vi "Sodium Boiler Model.vi"(5 "Heated Coolant Input (mB/t)":u32, 7 "Superheating Elements":u32=3 min=1 max=70 step=1, 8 "Steam Cavity Height (m)":u32, 9 "Water Cavity Height (m)":u32, 10 "Length (m)":u32=3 min=3 max=18 step=1, 11 "Width (m)":u32=4 min=3 max=18 step=1) -> ()   [LabVIEW 2023]
panel:
  out "Steam Tubes Required":u32=4 min=4 max=18 step=1
  out "Status":bool
  out "Water Demand (mB/t)":u32
  out "Boil Rate (mB/t)":dbl(slide) scale=0.0..9600000.0 scale format="%#_6f"
  out "Sodium Loops Required":u32=4 min=4 max=18 step=1
  out "Water Pipes Required":u32=4 min=4 max=18 step=1
  out "Steam Output (mB/t)":u32
  out "Coolant Output (mB/t)":u32
  out "Maximum Boil Rate (mB/t)":u32=4 min=4 max=18 step=1
  out "Coolant Tank (mB)":u32
  out "Steam Tank (mB)":u32
  out "Pressure Dispersers":u32=4 min=4 max=18 step=1
  out "Heated Coolant Tank (mB)":u32
  out "Water Tank (mB)":u32
  out "Volume (m³)":u32
  out "Height (m)":u32=4 min=4 max=18 step=1
  # "Thermoelectric Boiler Properties"
  # "Note: The boiler's heated coolant tank size must be about twice the size of the\nreactor's coolant tank, with as much coolant buffered in the coolant return tube\nand as much water as the water tank's capacity buffered in the water return tubes."
  # "Thermoelectric Boiler Operation"
  # "+1 for heating elements"
  # "+1 for dispersers"
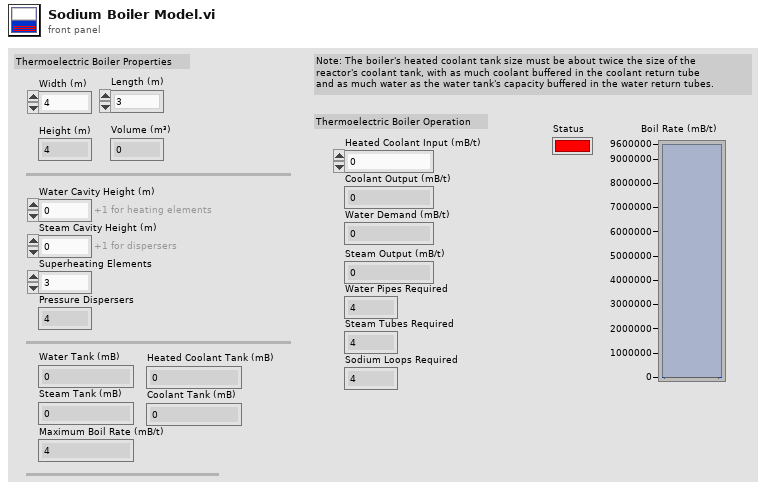
[diagram p1: front panel]
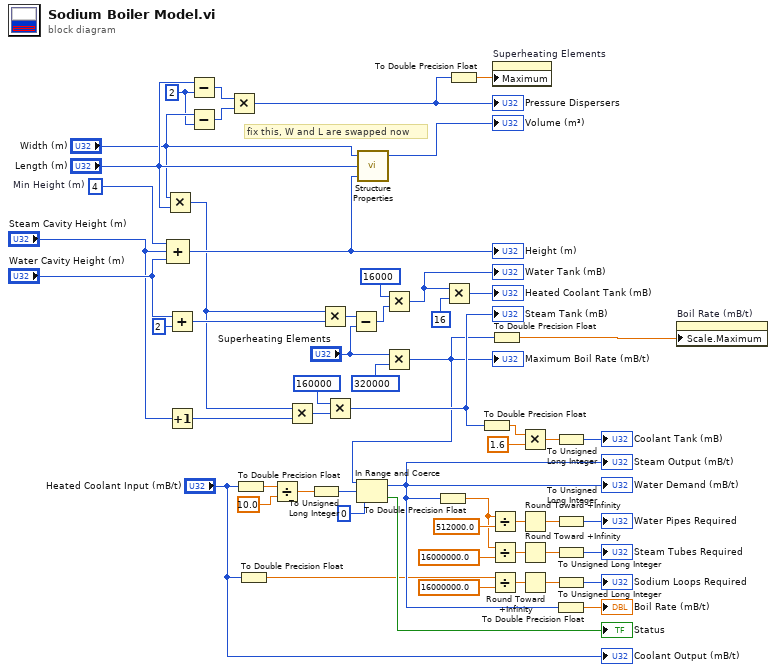
[diagram p0: block diagram]
diagram:
  w46 = u32 2 ("y")
  w55 = u32 4  # Min Height (m)
  # "fix this, W and L are swapped now"
  n1 = Multiply(x="Width (m)", y="Length (m)") -> (x*y=w32:u32)
  n2 = Compound Arithmetic op=ADD(w55, "Steam Cavity Height (m)", "Water Cavity Height (m)") -> (w54:u32)
  "Height (m)" <- w54
  n3 = Add(x="Water Cavity Height (m)", y=u32 2) -> (x+y=w33:u32)
  n4 = Increment(x="Steam Cavity Height (m)") -> (x+1=w31:u32)
  n5 = Subtract(x="Length (m)", y=w46) -> (x-y=w45:u32)
  n6 = Subtract(x="Width (m)", y=w46) -> (x-y=w44:u32)
  n7 = Multiply(x=w45, y=w44) -> (x*y=w2:u32)
  "Pressure Dispersers" <- w2
  n8 = To Double Precision Float(number="Heated Coolant Input (mB/t)") -> (double precision float=w19:dbl)
  n9 = To Double Precision Float(number="Heated Coolant Input (mB/t)") -> (double precision float=w9:dbl)
  n10 = Divide(x=w19, y=10.0) -> (x/y=w20:dbl)
  n11 = Multiply(x=w32, y=w31) -> (x*y=w38:u32)
  n12 = To Unsigned Long Integer(number=w20) -> (unsigned 32bit integer=w17:u32)
  n13 = Multiply(x=w32, y=w33) -> (x*y=w51:u32)
  n14 = Multiply(x=u32 160000 ("y"), y=w38) -> (x*y=w15:u32)
  "Steam Tank (mB)" <- w15
  n15 = Subtract(x=w51, y="Superheating Elements") -> (x-y=w49:u32)
  n16 = call "Structure Properties.vi"("Length"="Width (m)", "Width"="Length (m)", "Height"=w54) -> ("Volume"=→"Volume (m³)":i32)  [unwired: 2 in, 4 out]
  n17 = Multiply(x=u32 16000 ("y"), y=w49) -> (x*y=w43:u32)
  "Water Tank (mB)" <- w43
  n18 = Multiply(x="Superheating Elements", y=u32 320000) -> (x*y=w13:u32)
  "Maximum Boil Rate (mB/t)" <- w13
  n19 = In Range and Coerce(upper limit=w13, x=w17, lower limit=u32 0) -> (coerced(x)=w11:u32, In Range?=→"Status":bool)
  "Steam Output (mB/t)" <- w11
  "Water Demand (mB/t)" <- w11
  n20 = To Double Precision Float(number=w11) -> (double precision float=w3:dbl)
  n21 = Multiply(x=w43, y=u32 16) -> (x*y=→"Heated Coolant Tank (mB)":u32)
  n22 = To Double Precision Float(number=w2) -> (double precision float=w1:dbl)
  n23 = To Double Precision Float(number=w15) -> (double precision float=w14:dbl)
  n24 = Divide(x=w3, y=512000.0) -> (x/y=w27:dbl)
  n25 = Divide(x=w3, y=16000000.0) -> (x/y=w5:dbl)
  n26 = Divide(x=w9, y=16000000.0) -> (x/y=w26:dbl)
  n27 = To Double Precision Float(number=w13) -> (double precision float=w12:dbl)
  n28 = property on="Superheating Elements" class="DigNum (strict)"("Maximum"=w1) -> ()  [unwired: 2 in, 2 out]
  n29 = Multiply(x=w14, y=1.6) -> (x*y=w36:dbl)
  n30 = Round Toward +Infinity(x=w27) -> (ceil(x): smallest int >= x=w25:dbl)
  n31 = Round Toward +Infinity(x=w5) -> (ceil(x): smallest int >= x=w6:dbl)
  n32 = Round Toward +Infinity(x=w26) -> (ceil(x): smallest int >= x=w24:dbl)
  n33 = To Unsigned Long Integer(number=w36) -> (unsigned 32bit integer=→"Coolant Tank (mB)":u32)
  n34 = To Unsigned Long Integer(number=w25) -> (unsigned 32bit integer=→"Water Pipes Required":u32)
  n35 = To Unsigned Long Integer(number=w6) -> (unsigned 32bit integer=→"Steam Tubes Required":u32)
  n36 = To Unsigned Long Integer(number=w24) -> (unsigned 32bit integer=→"Sodium Loops Required":u32)
  n37 = To Double Precision Float(number=w11) -> (double precision float=→"Boil Rate (mB/t)":dbl)
  n38 = property on="Boil Rate (mB/t)" class="Slide (strict)"("Scale.Maximum"=w12) -> ()  [unwired: 2 in, 2 out]
  "Coolant Output (mB/t)" <- "Heated Coolant Input (mB/t)"
